vi "Send Send Direct Message.vi"(8 "error in (no error)":errorcluster, 10 "Message":T1, 11 "Chat Window UI Controller in":refnum<class "Chat Window UI Controller.lvclass">) -> (0 "error out":errorcluster, 3 "Chat Window UI Controller out":refnum<class "Chat Window UI Controller.lvclass">)   [LabVIEW 2020, in "Chat Window UI Controller.lvlib" / "Chat Window UI Controller.lvclass"]
uses:
  Chat Window UI Controller.lvclass
  C:/Program Files/National Instruments/LabVIEW 2020/vi.lib/ActorFramework/Actor/Actor.lvclass
  Controls/Message Control.ctl
  Event-Source-Actor/Data Interface/Message Data/Message Data.lvclass
  C:/Users/huipeng8/Desktop/SubPanel-Actor-Framework-master/Event-Source-Actor/Source/Template Source/Event Data/Event Data.lvclass
  <vilib>/ActorFramework/Actor/Actor.lvclass/Actor.ctl
  <vilib>/ActorFramework/Message Enqueuer/Message Enqueuer.lvclass/Message Enqueuer.ctl
  Chat Window UI Controller.lvclass/Chat Window UI Controller.ctl
  SubPanel-Actor-Framework-master/Event-Source-Actor/Source/Template Source/Event Source Messages/Generate Event Msg/Generate Event Msg.lvclass/Generate Event Msg.ctl
  <vilib>/ActorFramework/Message Enqueuer/Init from Existing Queue.vi
  <vilib>/ActorFramework/Message Enqueuer/Enqueue.vi
  SubPanel-Actor-Framework-master/Event-Source-Actor/Source/Template Source/Event Source Messages/Generate Event Msg/Generate Event Msg.lvclass
  C:/Program Files/National Instruments/LabVIEW 2020/vi.lib/ActorFramework/Message/Message.lvclass
  <vilib>/ActorFramework/Message Priority Queue/Priority Enqueue.vi
  <vilib>/ActorFramework/Message Enqueuer/Message Enqueuer.lvclass
  <vilib>/ActorFramework/Actor/Actor.lvclass
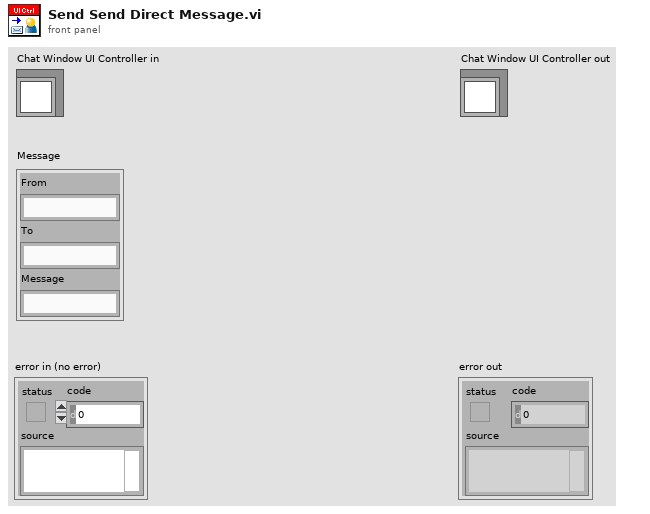
[diagram p1: front panel]
types:
  T1 = typedef "Message Control.ctl" = cluster{"From":string, "To":string, "Message":string}
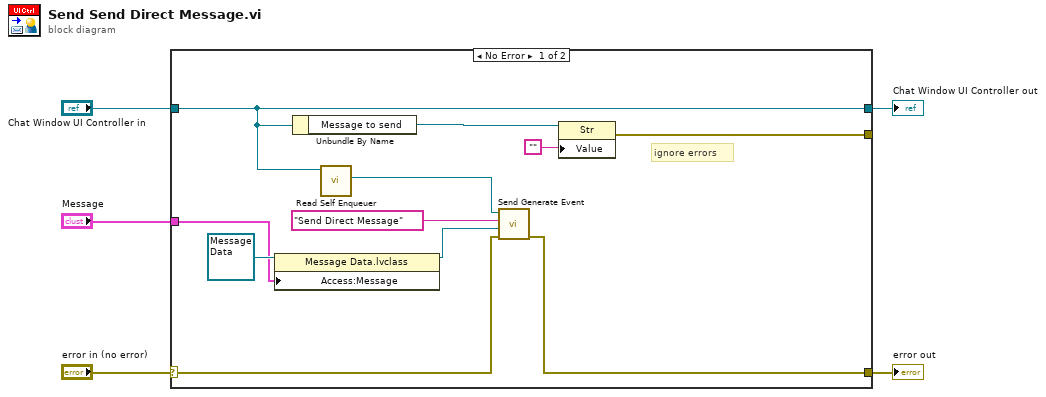
[diagram p0: block diagram]
diagram:
  n1 = case shown="No Error" "error in (no error)" {
    selector: "error in (no error)" -> [w9 w18]
    tunnel: [w8 w18] -> w4
    tunnel: [w16 w17] -> w2
    tunnel: "Chat Window UI Controller in" -> [w16 w17]
    tunnel: "Message" -> [w6 _]
    tunnel: [w13 _] -> _
    frame No Error {
      # "ignore errors"
      n2 = property class="Message Data.lvclass"(reference=refnum<class "Message Data.lvclass"> refnum ("Message Data.lvclass"), "Access:Message"=w6) -> (reference out=w10:refnum<class "Message Data.lvclass">)  [unwired: 1 in, 1 out]
      n3 = Unbundle By Name(w16) -> ("Message to send"=w15:refnum<vi>)
      n4 = call <vilib>:"Read Self Enqueuer.vi"("Actor"=w16) -> ("Self Enqueuer"=w7:refnum<class "Message Enqueuer.lvclass">)  [unwired: 10 in]
      n5 = call "Send Generate Event.vi"("error in"=w9, "Event Data"=w10, "Event Name"="Send Direct Message", "Message Enqueuer"=w7) -> ("error out"=w8:errorcluster)  [unwired: 6 in, 1 out]
      n6 = property class="Str"(reference=w15, "Value"="") -> (error out=w13:errorcluster)  [unwired: 1 in, 1 out]
    }
    frame Error {
    }
  }
  "error out" <- w4
  "Chat Window UI Controller out" <- w2
